vi "Test_UART.vi"() -> ()   [LabVIEW 2019]
uses:
  <vilib>/myRIO/Instrument Drivers/Onboard IO/UART/typedef/VISA Configuration.ctl
  <vilib>/Instr/_visa.llb/VISA Configure Serial Port (Instr).vi
  <vilib>/myRIO/Express VI/Onboard IO/UART/UART Express VI.xnode
  <vilib>/myRIO/Instrument Drivers/Onboard IO/UART/UART.lvlib
panel:
  in  "stop":bool
  in  "Servo_Gripper":dbl
  in  "Motor_Riel":dbl
  in  "Motor_Izquierdo":dbl
  in  "Motor_Derecho":dbl
  out "Trama de envío":string
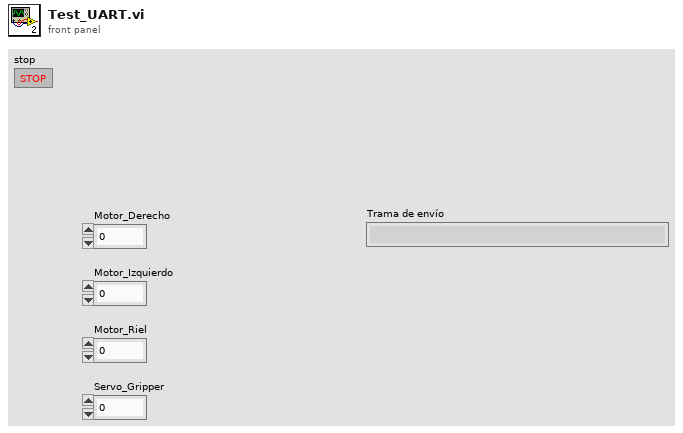
[diagram p1: front panel]
types:
  T1 = typedef "UART.lvlib/VISA Configuration.ctl" = cluster{"baud rate (9600)":u32, "data bits (8)":u16, "parity (0:none)":enum16{"None", "Odd", "Even", "Mark", "Space"}, "stop bits (10: 1 bit)":u16, "flow control (0:none)":u16, "termination char\n(0xA = '\\n' = LF) ":u8, "Enable Termination\nChar (T)":bool, "timeout (10sec)":u32}
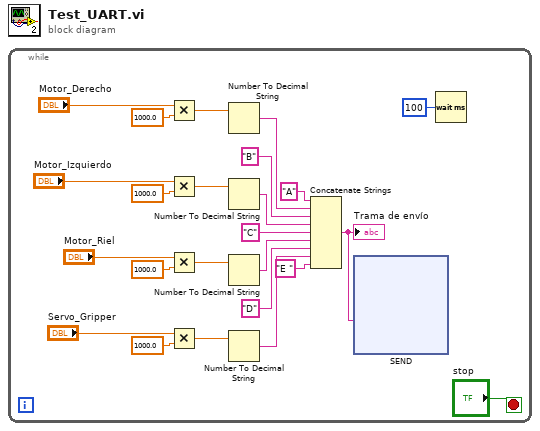
[diagram p0: block diagram]
diagram:
  n1 = while {
    stop <- "stop" stop-if-true
    n2 = Multiply(x="Motor_Derecho", y=1000.0) -> (x*y=w14:dbl)
    n3 = Multiply(x="Motor_Izquierdo", y=1000.0) -> (x*y=w8:dbl)
    n4 = Multiply(x="Motor_Riel", y=1000.0) -> (x*y=w7:dbl)
    n5 = Multiply(x="Servo_Gripper", y=1000.0) -> (x*y=w9:dbl)
    n6 = Number To Decimal String(number=w14) -> (decimal integer string=w16:string)  [unwired: 1 in]
    n7 = Number To Decimal String(number=w8) -> (decimal integer string=w18:string)  [unwired: 1 in]
    n8 = Number To Decimal String(number=w7) -> (decimal integer string=w20:string)  [unwired: 1 in]
    n9 = Number To Decimal String(number=w9) -> (decimal integer string=w23:string)  [unwired: 1 in]
    n10 = Concatenate Strings("A" ("string"), w16, "B" ("string"), w18, "C" ("string"), w20, "D" ("string"), w23, "E " ("string")) -> (w3:string)
    "Trama de envío" <- w3
    n11 = xnode "SEND"("Characters to Write"=w3) -> ()  [unwired: 1 in, 2 out]
    n12 = Wait (ms)(milliseconds to wait=u32 100) -> ()  [unwired: 1 out]
  }
